vi "clearJuicer.vi"(8 "error in (no error)":errorcluster, 11 "Juicer in":refnum<class "Juicer.lvclass">) -> (0 "error out":errorcluster, 3 "Juicer out":refnum<class "Juicer.lvclass">)   [LabVIEW 2014, in "Juicer.lvclass"]
uses:
  Juicer.lvclass
  Juicer.lvclass/Juicer.ctl
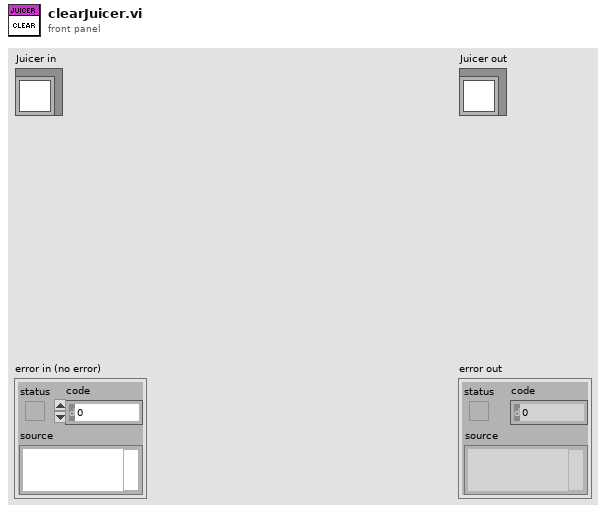
[diagram p1: front panel]
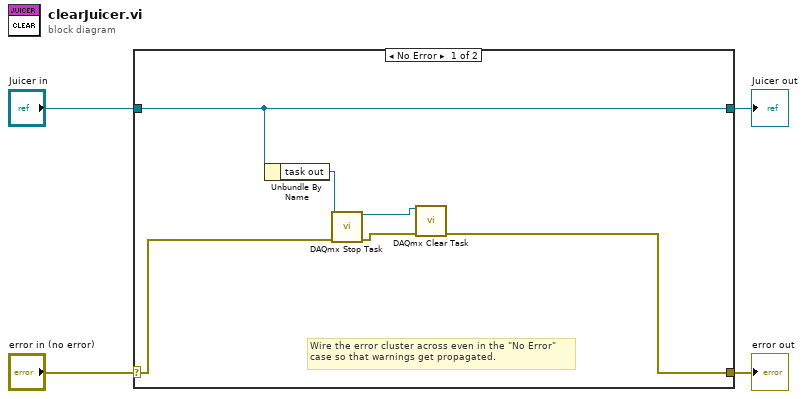
[diagram p0: block diagram]
diagram:
  n1 = case shown="No Error" "error in (no error)" {
    selector: "error in (no error)" -> [w5 w12]
    tunnel: [w6 w12] -> w3
    tunnel: [w10 w11] -> w1
    tunnel: "Juicer in" -> [w10 w11]
    frame No Error {
      # "Wire the error cluster across even in the \"No Error\"\ncase so that warnings get propagated."
      n2 = Unbundle By Name(w10) -> ("task out"=w9:refnum<k21>)
      n3 = call <vilib>:"DAQmx Stop Task.vi"("task/channels in"=w9, "error in"=w5) -> ("task out"=w8:refnum<k21>, "error out"=w7:errorcluster)  [unwired: 12 in]
      n4 = call <vilib>:"DAQmx Clear Task.vi"("task in"=w8, "error in"=w7) -> ("error out"=w6:errorcluster)  [unwired: 13 in]
    }
    frame Error {
    }
  }
  "error out" <- w3
  "Juicer out" <- w1
